vi "Calculate Index Array.vi"(8 "error in (no error)":errorcluster, 10 "3D Comet Datatype.lvclass in":refnum<class "3D Comet Datatype.lvclass">, 11 "Plot Representation In":T1) -> (0 "error out":errorcluster, 2 "3D Comet Datatype.lvclass out":refnum<class "3D Comet Datatype.lvclass">, 3 "Plot Representation Out":T1)   [LabVIEW 2020, in "3D Comet Datatype.lvclass"]
uses:
  <vilib>/Math Plots/3D Math Plots/3D Comet/3D Comet Datatype/3D Comet Datatype.lvclass
  <vilib>/Math Plots/3D Math Plots/3D Plot/3D Plot/Typedef/Plot Representation.ctl
  <vilib>/Math Plots/3D Math Plots/3D Plot/3D Plot/Typedef/Range Clusters.ctl
  <vilib>/Math Plots/3D Math Plots/3D Plot/3D Plot/Typedef/Mesh Data.ctl
  <vilib>/Math Plots/3D Math Plots/3D Plot/3D Plot/3D Plot.lvclass
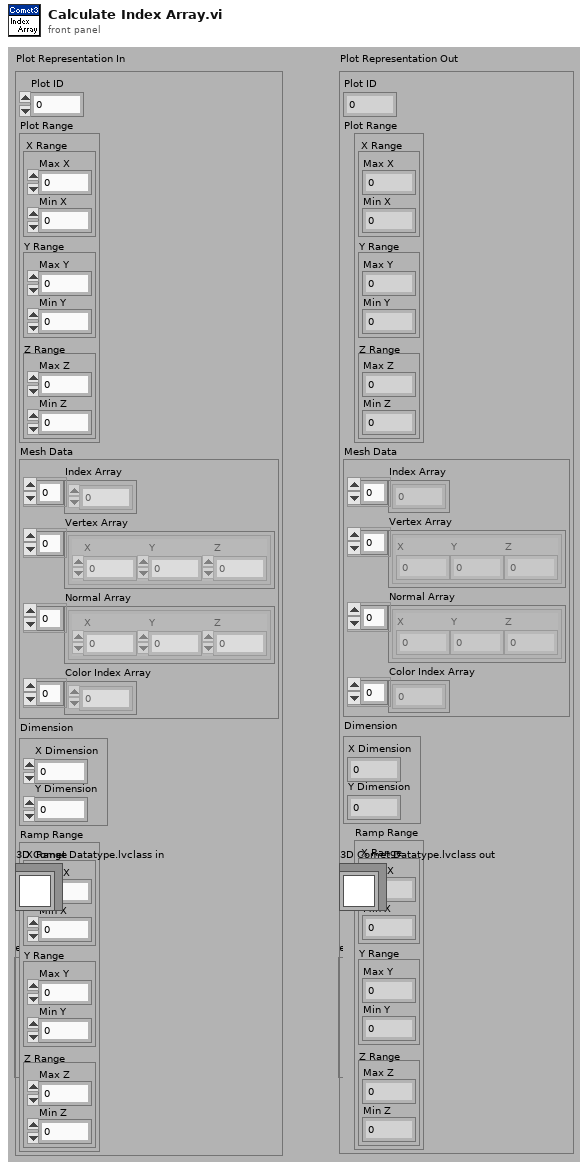
[diagram p1: front panel]
types:
  T1 = typedef "3D Plot.lvclass/Plot Representation.ctl" = cluster{"Plot ID":i32, "Plot Range":T2, "Mesh Data":T3, "Dimension":cluster{"X Dimension":i32, "Y Dimension":i32}, "Ramp Range":T2}
  T2 = typedef "3D Plot.lvclass/Range Clusters.ctl" = cluster{"X Range":cluster{"Max X":sgl, "Min X":sgl}, "Y Range":cluster{"Max Y":sgl, "Min Y":sgl}, "Z Range":cluster{"Max Z":sgl, "Min Z":sgl}}
  T3 = typedef "3D Plot.lvclass/Mesh Data.ctl" = cluster{"Index Array":u32[], "Vertex Array":cluster{"X":sgl, "Y":sgl, "Z":sgl}[], "Normal Array":cluster{"X":sgl, "Y":sgl, "Z":sgl}[], "Color Index Array":i32[]}
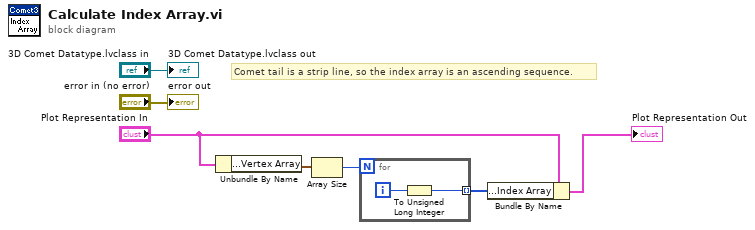
[diagram p0: block diagram]
diagram:
  # "Comet tail is a strip line, so the index array is an ascending sequence."
  n1 = Unbundle By Name("Plot Representation In") -> ("Mesh Data.Vertex Array"=w3:cluster{"X":sgl, "Y":sgl, "Z":sgl}[])
  n2 = Array Size(array=w3) -> (size(s)=w2:i32)
  n3 = for {
    N: w2 -> [_]
    tunnel: [w8] -> w1 mode=indexing
    i -> [w9]
    n4 = To Unsigned Long Integer(number=w9) -> (unsigned 32bit integer=w8:u32)
  }
  n5 = Bundle By Name(cluster="Plot Representation In", "Mesh Data.Index Array"=w1) -> (→"Plot Representation Out":T1)
  "error out" <- "error in (no error)"
  "3D Comet Datatype.lvclass out" <- "3D Comet Datatype.lvclass in"
